vi "MultiPlotting_6Plot_DPVer1.0.vi"(0 "2D-DataIn":dbl[][](array[numeric]), 1 "DataDisplay Ref Array":refnum<vi>[](array[refnum]), 3 "DisplayControl":T2 {"Scale" items=["L", "R"]; "Y - axes"."Y 6" items=["", "Realtime_sec", "Intervaltime_sec", "OscillatorFreq_Hz", "SR7265_1_Vx_Volt", "SR7265_1_Vy_Volt", "Ohm"]; "Y - axes"."Y 5" items=["", "Realtime_sec", "Intervaltime_sec", "OscillatorFreq_Hz", "SR7265_1_Vx_Volt", "SR7265_1_Vy_Volt", "Ohm"]; "Y - axes"."Y 4" items=["", "Realtime_sec", "Intervaltime_sec", "OscillatorFreq_Hz", "SR7265_1_Vx_Volt", "SR7265_1_Vy_Volt", "Ohm"]; "Y - axes"."Y 3" items=["", "Realtime_sec", "Intervaltime_sec", "OscillatorFreq_Hz", "SR7265_1_Vx_Volt", "SR7265_1_Vy_Volt", "Ohm"]; "Y - axes"."Y 2" items=["", "Realtime_sec", "Intervaltime_sec", "OscillatorFreq_Hz", "SR7265_1_Vx_Volt", "SR7265_1_Vy_Volt", "Ohm"]; "Y - axes"."Y 1" items=["", "Realtime_sec", "Intervaltime_sec", "OscillatorFreq_Hz", "SR7265_1_Vx_Volt", "SR7265_1_Vy_Volt", "Ohm"]; "X - axis" items=["Realtime_sec", "Intervaltime_sec", "OscillatorFreq_Hz", "SR7265_1_Vx_Volt", "SR7265_1_Vy_Volt", "Ohm"]}) -> (5 "DataDisplay":T1 {"X" format="%#_6e"; "Y 5" format="%#_6e"; "Y 4" format="%#_6e"; "Y 3" format="%#_6e"; "Y 6" format="%#_6e"; "Y 2" format="%#_6e"; "Y 1" format="%#_6e"}, 7 "XY Graph":cluster{"DataOut":dbl[], "DataOut":dbl[]}[](graph))   [LabVIEW 2012]
doc: "2D array input, and select 6 colums to plot XY graph. This subVI only support 6 plotting lines. If more than 6 plottings are required, please increase the number of Y-axes control ring in DisplayControl."
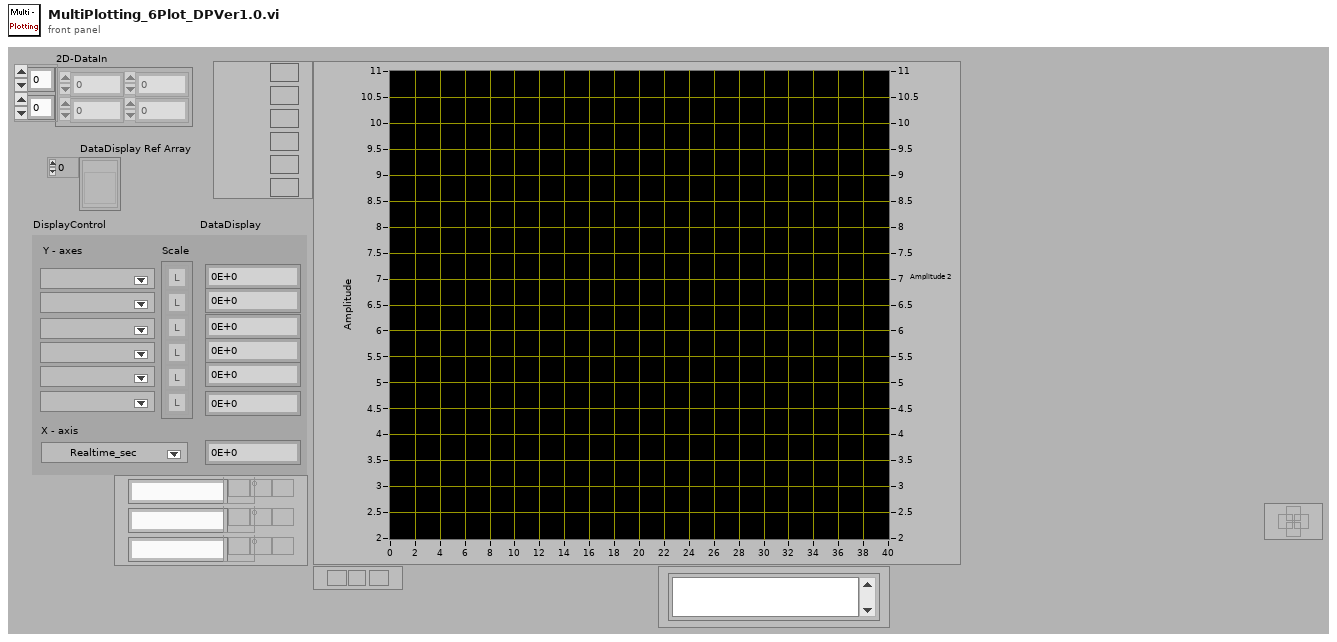
[diagram p1: front panel]
types:
  T1 = cluster{"X":dbl, "Y 1":dbl, "Y 2":dbl, "Y 3":dbl, "Y 4":dbl, "Y 5":dbl, "Y 6":dbl}
  T2 = cluster{"X - axis":u8, "Y - axes":cluster{"Y 1":u8, "Y 2":u8, "Y 3":u8, "Y 4":u8, "Y 5":u8, "Y 6":u8}, "Scale":u16[]}
  T3 = cluster{"Y 1":u8, "Y 2":u8, "Y 3":u8, "Y 4":u8, "Y 5":u8, "Y 6":u8}
  T4 = cluster{"[0]":dbl, "[1]":dbl, "[2]":dbl, "[3]":dbl, "[4]":dbl, "[5]":dbl, "[6]":dbl}
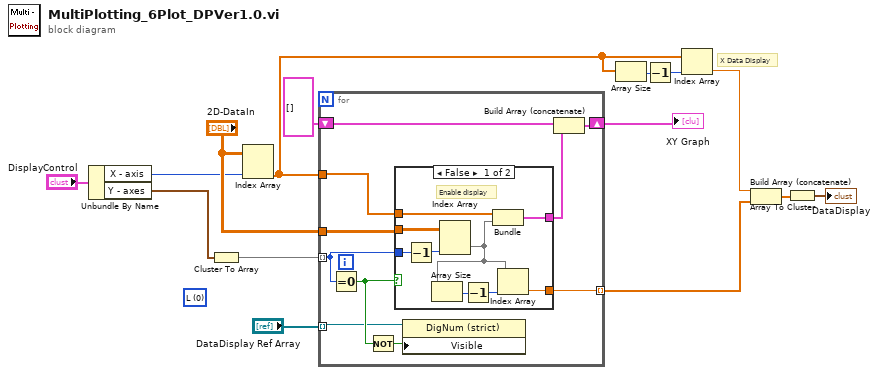
[diagram p0: block diagram]
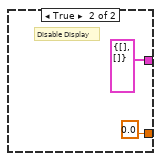
[diagram p2: hidden frame]
diagram:
  (unwired) u16 0 items=["L", "R"] ("Y-axes slector 2")
  # "X Data Display"
  n1 = Unbundle By Name("DisplayControl") -> ("X - axis"=w12:u8, "Y - axes"=w14:T3)
  n2 = Cluster To Array(cluster=w14) -> (array=w15:u8[])
  n3 = Index Array(array="2D-DataIn", index (col)=w12) -> (element=w6:dbl[])  [unwired: 1 in]
  n4 = for {
    tunnel: w15 -> [w21] mode=indexing
    shift-right: [w24] -> w10
    shift-left: cluster{"DataOut":dbl[], "DataOut":dbl[]}[] [] -> [w23]
    tunnel: w6 -> [w20]
    tunnel: "2D-DataIn" -> [w22]
    tunnel: [w19] -> w4 mode=indexing
    tunnel: "DataDisplay Ref Array" -> [w16] mode=indexing
    n5 = Equal To 0?(x=w21) -> (x = 0?=w18:bool)
    n6 = Not(x=w18) -> (.not. x?=w17:bool)
    n7 = case shown="False" w18 {
      tunnel: w22 -> [w34 _]
      tunnel: w20 -> [w33 _]
      tunnel: [w32 cluster{"DataOut":dbl[], "DataOut":dbl[]} {"DataOut"=[], "DataOut"=[]}] -> w25
      tunnel: w21 -> [w31 _]
      tunnel: [w26 0.0] -> w19
      frame False {
        # "Enable display"
        n8 = Decrement(x=w31) -> (x-1=w30:u8)
        n9 = Index Array(array=w34, index (col)=w30) -> (element=w27:dbl[])  [unwired: 1 in]
        n10 = Array Size(array=w27) -> (size(s)=w28:i32)
        n11 = Decrement(x=w28) -> (x-1=w29:i32)
        n12 = Bundle("2D-DataIn"=w33, "2D-DataIn"=w27) -> (w32:cluster{"2D-DataIn":dbl[], "2D-DataIn":dbl[]})  [unwired: 1 in]
        n13 = Index Array(array=w27, index=w29) -> (element=w26:dbl)
      }
      frame True {
        # "Disable Display"
      }
    }
    n14 = property class="DigNum (strict)"(reference=w16, "Visible"=w17) -> ()  [unwired: 1 in, 2 out]
    n15 = Build Array (concatenate)(w23, w25) -> (w24:cluster{"DataOut":dbl[], "DataOut":dbl[]}[])
  }
  "XY Graph" <- w10
  n16 = Array Size(array=w6) -> (size(s)=w7:i32)
  n17 = Decrement(x=w7) -> (x-1=w8:i32)
  n18 = Index Array(array=w6, index=w8) -> (element=w5:dbl)
  n19 = Build Array (concatenate)(w5, w4) -> (w3:dbl[])
  n20 = Array To Cluster(array=w3) -> (cluster=→"DataDisplay":T4)
